vi "VCI_Transmit.vi"(0 "DevType":u32=4, 1 "指令名":dbl, 5 "DevIndex":u32, 9 "CANIndex":u32, 11 "Len":u32=1, 12 "参数1":dbl format="%#_f", 13 "参数2":dbl, 14 "参数3":dbl) -> (4 "DevType 2":u32=4, 6 "DevIndex 2":u32, 10 "CANIndex 2":u32, 15 "发送的帧数":u32=1)   [LabVIEW 2014]
uses:
  ControlCAN.dll
panel:
  out "VCI_CAN_OBJ 2":T1={"ID"=0, "TimeStamp"=0, "TimeFlag"=0, "SendType"=2, "RemoteFlag"=0, "ExternFlag"=0, "DataLen"=0, "Data 0"=0, "Data 1"=1, "Data 2"=0, "Data 3"=0, "Data 4"=0, "Data 5"=0, "Data 6"=0, "Data 7"=0, "Reserved 0"=0, "Reserved 1"=0, "Reserved 2"=0}
  out "Len 2":u32=1
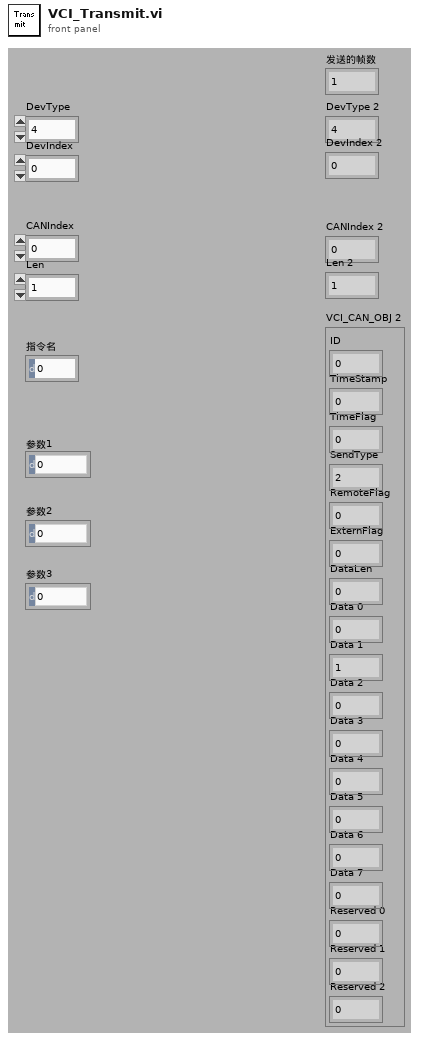
[diagram p1: front panel]
types:
  T1 = cluster{"ID":u32, "TimeStamp":u32, "TimeFlag":u8, "SendType":u8, "RemoteFlag":u8, "ExternFlag":u8, "DataLen":u8, "Data 0":u8, "Data 1":u8, "Data 2":u8, "Data 3":u8, "Data 4":u8, "Data 5":u8, "Data 6":u8, "Data 7":u8, "Reserved 0":u8, "Reserved 1":u8, "Reserved 2":u8}
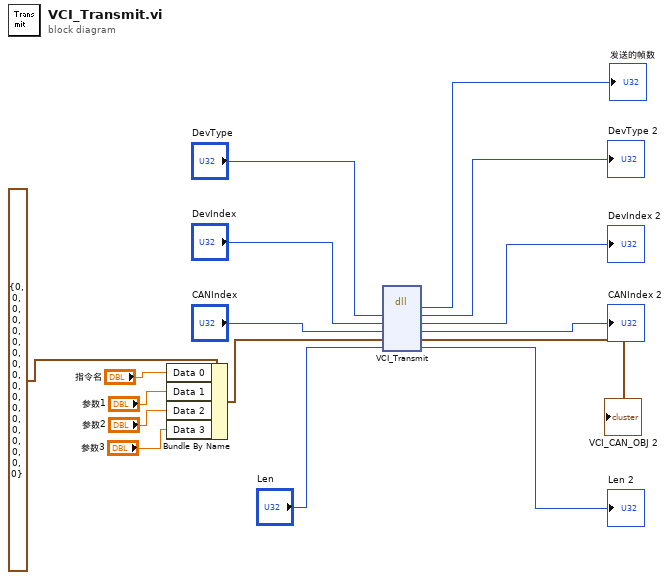
[diagram p0: block diagram]
diagram:
  n1 = Bundle By Name(cluster=T1 {"ID"=0, "TimeStamp"=0, "TimeFlag"=0, "SendType"=0, "RemoteFlag"=0, "ExternFlag"=0, "DataLen"=0, "Data 0"=0, "Data 1"=0, "Data 2"=0, "Data 3"=0, "Data 4"=0, "Data 5"=0, "Data 6"=0, "Data 7"=0, "Reserved 0"=0, "Reserved 1"=0, "Reserved 2"=0} ("VCI_CAN_OBJ 2"), "Data 0"="指令名", "Data 1"="参数1", "Data 2"="参数2", "Data 3"="参数3") -> (w1:T1)
  n2 = dll-call lib="PTH22abs D\tDocuments\tCan总线canControlCAN.dll" fn="VCI_Transmit"("DevType"="DevType", "DevIndex"="DevIndex", "CANIndex"="CANIndex", "VCI_CAN_OBJ 2"=w1, "Len"="Len") -> ("发送的帧数"=→"发送的帧数":u32, "DevType"=→"DevType 2":u32, "DevIndex"=→"DevIndex 2":u32, "CANIndex"=→"CANIndex 2":u32, "VCI_CAN_OBJ 2"=→"VCI_CAN_OBJ 2":T1, "Len"=→"Len 2":u32)  [unwired: 3 in, 2 out]
